vi "Set Elevation.vi"(0 "GMaps API in":refnum<class "GMaps API.lvclass">, 1 "Latitude":string, 2 "Longitude":string=" ", 5 "error in (no error)":errorcluster) -> (14 "GMaps API out":refnum<class "GMaps API.lvclass">, 19 "error out":errorcluster)   [LabVIEW 2016, in "GMaps API.lvclass"]
doc: "Sets elevation for all locations on the surface of the earth."
uses:
  GMaps API.lvclass
  GMaps API.lvclass/GMaps API.ctl
  <vilib>/regexp/Match Regular Expression.xnode
  <vilib>/httpClient/LabVIEWHTTPClient.lvlib
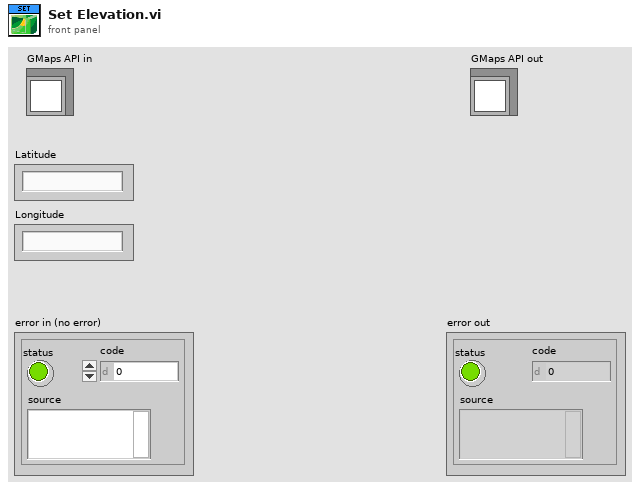
[diagram p1: front panel]
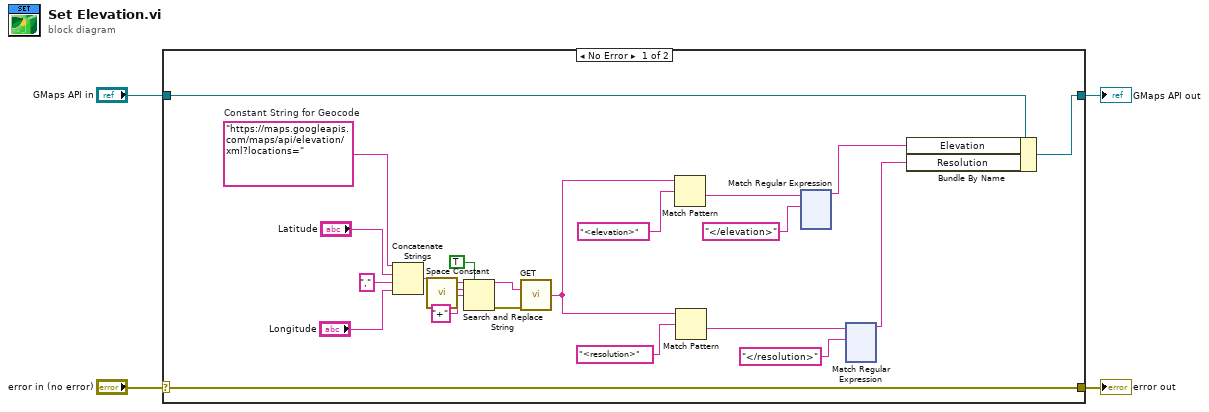
[diagram p0: block diagram]
diagram:
  n1 = case shown="No Error" "error in (no error)" {
    selector: "error in (no error)" -> [w26 w256]
    tunnel: [w26 w256] -> w3
    tunnel: [w24 w255] -> w1
    tunnel: "GMaps API in" -> [w25 w255]
    frame No Error {
      w20 = "https://maps.googleapis.com/maps/api/elevation/xml?locations="  # Constant String for Geocode
      n2 = Concatenate Strings(w20, "Latitude", "," ("string"), "Longitude") -> (w7:string)
      n3 = call <vilib>:"Space Constant.vi"() -> ("String"=w18:string)
      n4 = Search and Replace String(replace all?=TRUE ("replace all? (F)"), input string=w7, search string=w18, replace string="+" ("replace string (\"\")")) -> (result string=w15:string, error out=w16:errorcluster)  [unwired: 4 in, 2 out]
      n5 = call <vilib>:"GET.vi"("url"=w15, "error in (no error)"=w16) -> ("body"=w11:string)  [unwired: 10 in, 3 out]
      n6 = Match Pattern(string=w11, regular expression="<elevation>") -> (after substring=w10:string)  [unwired: 4 out]
      n7 = Match Pattern(string=w11, regular expression="<resolution>" ("Directly Before Latitude info")) -> (after substring=w9:string)  [unwired: 4 out]
      n8 = xnode "Match Regular Expression"("input string"=w10, "regular expression"="</elevation>") -> ("before match"=w5:string)  [unwired: 4 in, 4 out]
      n9 = xnode "Match Regular Expression"("input string"=w9, "regular expression"="</resolution>" ("Directly After Latitude info")) -> ("before match"=w6:string)  [unwired: 4 in, 4 out]
      n10 = Bundle By Name(cluster=w25, "Elevation"=w5, "Resolution"=w6) -> (w24:refnum<class "GMaps API.lvclass">)
    }
    frame Error {
    }
  }
  "error out" <- w3
  "GMaps API out" <- w1
